vi "Write Error.vi"(8 "error in (no error)":errorcluster, 10 "Error":errorcluster, 11 "LHW-Data in":refnum<class "LHW-Data.lvclass">) -> (0 "error out":errorcluster, 3 "LHW-Data out":refnum<class "LHW-Data.lvclass">)   [LabVIEW 2016, in "LHW-Data.lvlib" / "LHW-Data.lvclass"]
doc: "Write error information to attribute."
uses:
  LHW-Data.lvclass
  LHW-Data.lvclass/LHW-Data.ctl
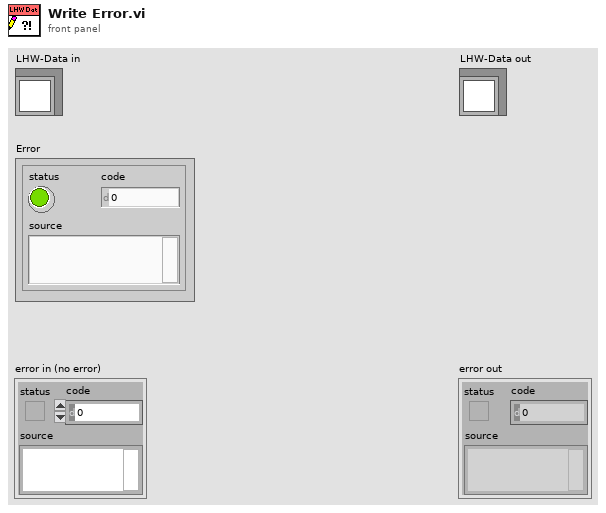
[diagram p1: front panel]
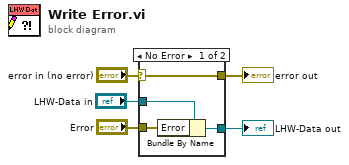
[diagram p0: block diagram]
diagram:
  n1 = case shown="No Error" "error in (no error)" {
    selector: "error in (no error)" -> [w9 w10]
    tunnel: [w9 w10] -> w4
    tunnel: [w7 w11] -> w2
    tunnel: "LHW-Data in" -> [w8 w11]
    tunnel: "Error" -> [w6 _]
    frame No Error {
      n2 = Bundle By Name(cluster=w8, "Error"=w6) -> (w7:refnum<class "LHW-Data.lvclass">)
    }
    frame Error {
    }
  }
  "error out" <- w4
  "LHW-Data out" <- w2
